vi "stop counter.vi"(7 "action":enum16{"init", "check"}(ring), 10 "stop counter control":T1={"counter (min)"=1600, "done"=FALSE, "everything to zero"=TRUE, "after (#min)"=1600.0, "to zero counter sec)"=85, "to zero start (sec)"=104}, 11 "seconds":i32=85) -> (2 "stop counter control out":T1={"counter (min)"=1600, "done"=FALSE, "everything to zero"=TRUE, "after (#min)"=1600.0, "to zero counter sec)"=85, "to zero start (sec)"=104}, 3 "done":bool)   [LabVIEW 2010]
uses:
  stop counter control.ctl
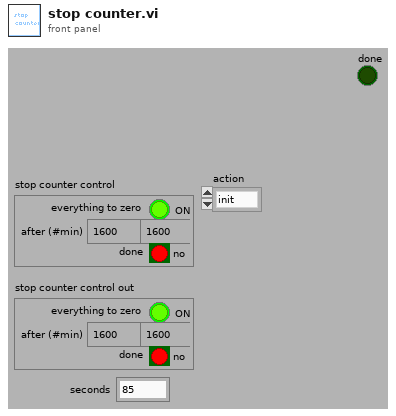
[diagram p1: front panel]
types:
  T1 = typedef "stop counter control.ctl" = cluster{"counter (min)":i32, "done":bool, "everything to zero":bool, "after (#min)":dbl, "to zero counter sec)":i32, "to zero start (sec)":i32}
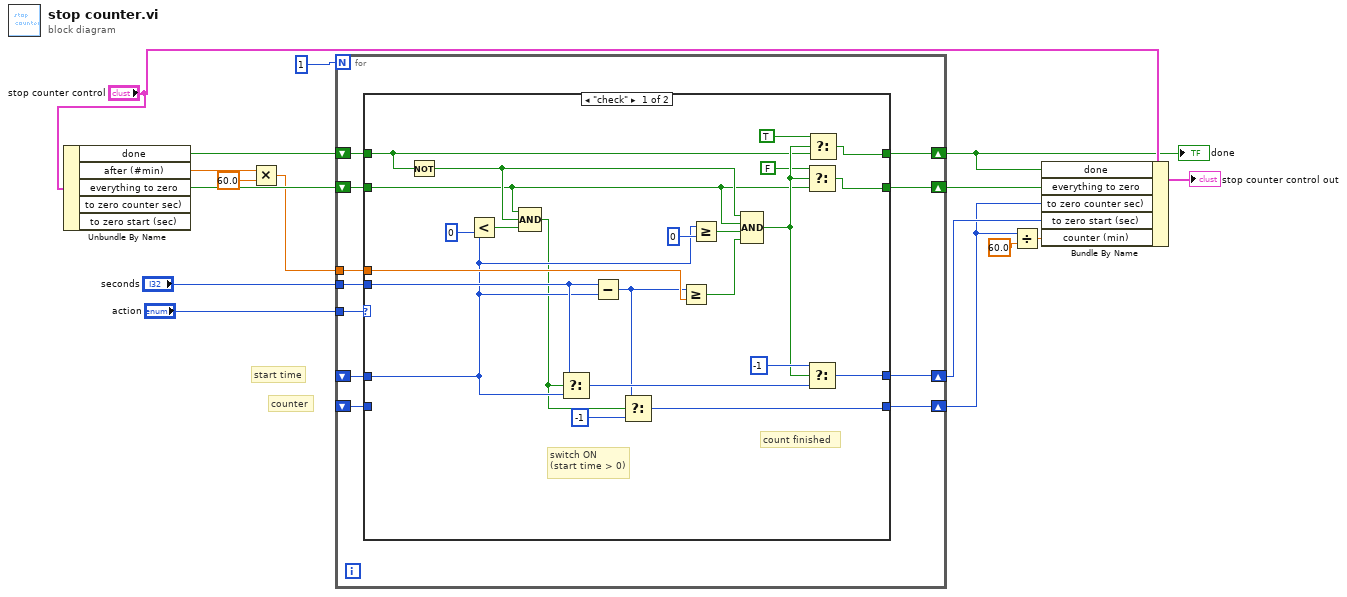
[diagram p0: block diagram]
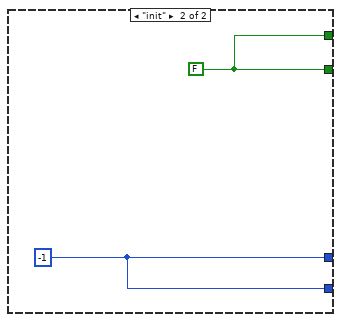
[diagram p2: hidden frame]
diagram:
  # "counter"
  # "start time"
  n1 = Unbundle By Name("stop counter control") -> ("done"=w12:bool, "after (#min)"=w11:dbl, "everything to zero"=w13:bool)  [unwired: 2 out]
  n2 = Multiply(x=w11, y=60.0) -> (x*y=w9:dbl)
  n3 = for {
    N: 1 -> [_]
    tunnel: "action" -> [w26]
    shift-right: [w23] -> w6
    shift-left: _ -> [w19]
    shift-right: [w24] -> w1
    shift-left: w13 -> [w25]
    shift-right: [w22] -> w5
    shift-left: _ -> [w17]
    shift-right: [w20] -> w2
    shift-left: w12 -> [w21]
    tunnel: "seconds" -> [w27]
    tunnel: w9 -> [w18]
    n4 = case shown="\"check\"" w26 {
      tunnel: w27 -> [w44 _]
      tunnel: [w28 w51] -> w24
      tunnel: w25 -> [w30 _]
      tunnel: [w40 w52] -> w23
      tunnel: [w36 w52] -> w22
      tunnel: w21 -> [w31 _]
      tunnel: [w29 w51] -> w20
      tunnel: w19 -> [w43 _]
      tunnel: w18 -> [w45 _]
      tunnel: w17 -> [_ _]
      frame "check" {
        # "count finished"
        # "switch ON\n(start time > 0)"
        n5 = Not(x=w31) -> (.not. x?=w46:bool)
        n6 = Less?(x=w43, y=0) -> (x < y?=w49:bool)
        n7 = Compound Arithmetic op=AND(w30, w46, w49) -> (w38:bool)
        n8 = Select(t=w44, s=w38, f=w43) -> (s? t:f=w41:i32)
        n9 = Subtract(x=w44, y=w43) -> (x-y=w39:i32)
        n10 = Select(t=w39, s=w38, f=-1) -> (s? t:f=w36:i32)
        n11 = Greater Or Equal?(x=w39, y=w45) -> (x >= y?=w42:bool)
        n12 = Greater Or Equal?(x=w43, y=0) -> (x >= y?=w47:bool)
        n13 = Compound Arithmetic op=AND(w46, w30, w47, w42) -> (w34:bool)
        n14 = Select(t=FALSE, s=w34, f=w30) -> (s? t:f=w28:bool)
        n15 = Select(t=-1, s=w34, f=w41) -> (s? t:f=w40:i32)
        n16 = Select(t=TRUE, s=w34, f=w31) -> (s? t:f=w29:bool)
      }
      frame "init" {
        w51 = FALSE
        w52 = -1
      }
    }
  }
  "done" <- w2
  n17 = Divide(x=w5, y=60.0) -> (x/y=w3:dbl)
  n18 = Bundle By Name(cluster="stop counter control", "done"=w2, "everything to zero"=w1, "to zero counter sec)"=w5, "to zero start (sec)"=w6, "counter (min)"=w3) -> (→"stop counter control out":T1)
